vi "Complex Back Transform Eigenvectors.vi"(6 "Scale":dbl[](array[numeric]), 7 "job":T1=3 items=["Neither Permuted nor Scaled", "Permuted but not Scaled", "Scaled but not Permuted", "Both Permuted and Scaled"], 8 "side":u16(ring) items=["Right Eigenvectors", "Left Eigenvectors"], 9 "index high":i32, 10 "index low":i32, 11 "Eigenvectors":T2) -> (0 "error":i32, 3 "Transformed Eigenvectors":T2)   [LabVIEW 2017, in "NI_AALPro.lvlib"]
doc: "Transforms the eigenvectors of a balanced matrix to those of the original matrix. Wire data to the <B>Eigenvectors</B> input to determine the polymorphic instance to use or manually select the instance."
uses:
  <vilib>/Analysis/NI_AALPro.lvlib
  <vilib>/Analysis/Matrix/Datatypes/ComplexMatrix.ctl
  <vilib>/Analysis/7linalg.llb/Matrix Balance Job.ctl
  <resource>/lvanlys.dll
  <vilib>/Analysis/Matrix/NI_Matrix.lvlib
panel:
  # "Transforms eigenvectors of a balanced matrix to those of the original nonsymmetric matrix"
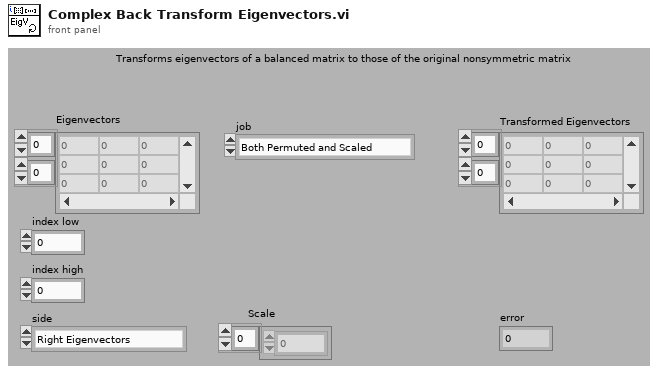
[diagram p1: front panel]
types:
  T1 = typedef "NI_AALPro.lvlib/Matrix Balance Job.ctl" = u16
  T2 = typedef "NI_Matrix.lvlib/ComplexMatrix.ctl" = cdb[][]
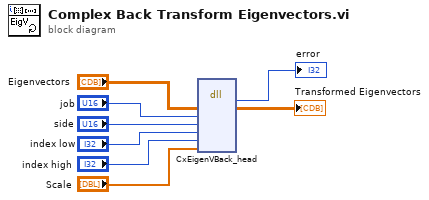
[diagram p0: block diagram]
diagram:
  n1 = dll-call lib="e:/builds/penguin/labview/branches/2017/dev/dist/resource/lvanlys.*" fn="CxEigenVBack_head"("Eigenvectors"="Eigenvectors", "job"="job", "side"="side", "ilo"="index low", "ihi"="index high", "Scale"="Scale") -> (→"error":i32, "Eigenvectors"=→"Transformed Eigenvectors":T2)  [unwired: 8 in, 2 out]
